vi "Read Current Message.vi"(8 "error in (no error)":errorcluster, 11 "System Log in":refnum<class "System Log.lvclass">) -> (0 "error out":errorcluster, 2 "Current Msgs":string[](array[string]), 3 "System Log out":refnum<class "System Log.lvclass">)   [LabVIEW 2016, in "System Log.lvclass"]
uses:
  System Log.lvclass
  System Log.lvclass/System Log.ctl
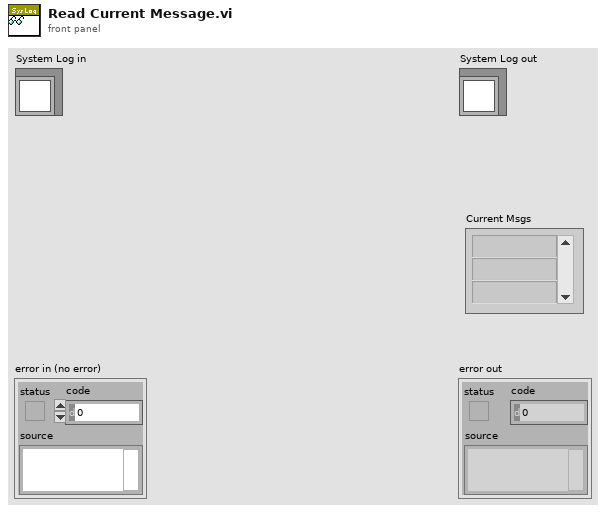
[diagram p1: front panel]
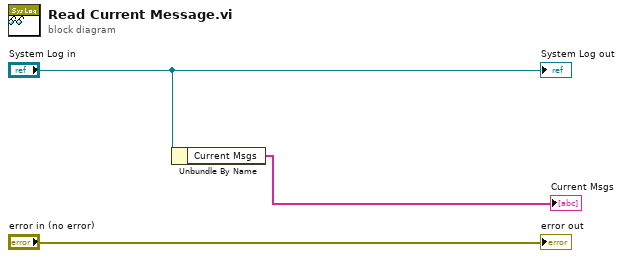
[diagram p0: block diagram]
diagram:
  n1 = Unbundle By Name("System Log in") -> ("Current Msgs"=→"Current Msgs":string[])
  "error out" <- "error in (no error)"
  "System Log out" <- "System Log in"
